vi "Settings.vi"(8 "error in":errorcluster, 10 "Main":T4={"Heat"={"KPтерм"=8.0, "TNтерм"=12.0, "KPниз"=4.0, "TNниз"=8.0, "COM ADC"="", "COM Termex"="", "KPдд"=4.0, "TNдд"=8.0, "Multiper"=1.0}, "Расчёты"={"Vm0"=8.0, "aa"=8.0, "bb"=8.0, "K0"=8.0, "A"=8.0, "B"=8.0}, "Видеосистема"=FALSE, "Anton Paar"={"IP adress"="192.168.0.110"}, "MIDA COM"="COM11"} caption="Настройки" {"Расчёты"."B" min=0.0 max=150.0 format="%.8f"; "Расчёты"."A" min=0.0 max=150.0 format="%.8f"; "Расчёты"."K0" min=0.0 max=150.0 format="%.2f"; "Расчёты"."bb" min=0.0 max=150.0 format="%.8f"; "Расчёты"."aa" min=0.0 max=150.0 format="%.8f"; "Расчёты"."Vm0" min=0.0 max=150.0 format="%.2f"; "Heat"."Multiper" min=0.0 max=150.0 format="%.2f"; "Heat"."TNдд" min=0.0 max=150.0 format="%.2f"; "Heat"."KPдд" min=0.0 max=150.0 format="%.2f"; "Heat"."TNниз" min=0.0 max=150.0 format="%.2f"; "Heat"."KPниз" min=0.0 max=150.0 format="%.2f"; "Heat"."TNтерм" min=0.0 max=150.0 format="%.2f"; "Heat"."KPтерм" min=0.0 max=150.0 format="%.2f"}) -> (0 "error out":errorcluster)   [LabVIEW 2023, in "Settings Master.lvlib"]
doc: "_____\nCreated using DQMH Event Scripter 6.1.0.128."
uses:
  Settings Master.lvlib
  Heat UI/Settings Type.ctl
  Drive/Calc_Type.ctl
  Menu/Setts.ctl
  Settings Argument--cluster.ctl
  Heat UI/Heat UI.lvlib
  Drive/Drive.lvlib
  Menu/Menu.lvlib
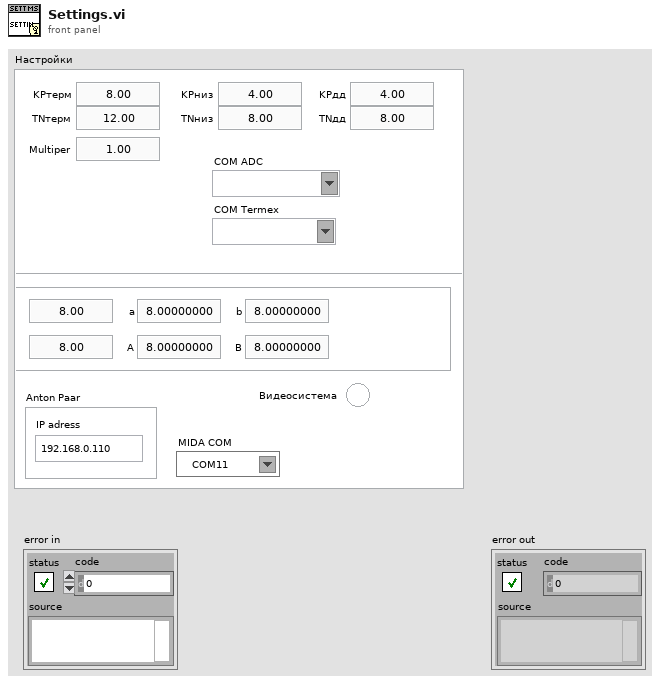
[diagram p1: front panel]
types:
  T1 = typedef "Heat UI.lvlib/Settings Type.ctl" = cluster{"KPтерм":dbl, "TNтерм":dbl, "KPниз":dbl, "TNниз":dbl, "COM ADC":refnum<visa-resource-name>, "COM Termex":refnum<visa-resource-name>, "KPдд":dbl, "TNдд":dbl, "Multiper":dbl}
  T2 = typedef "Drive.lvlib/Calc_Type.ctl" = cluster{"Vm0":dbl, "aa":dbl, "bb":dbl, "K0":dbl, "A":dbl, "B":dbl}
  T3 = typedef "Menu.lvlib/Setts.ctl" = cluster{"IP adress":string}
  T4 = cluster{"Heat":T1, "Расчёты":T2, "Видеосистема":bool, "Anton Paar":T3, "MIDA COM":refnum<visa-resource-name>}
  T5 = typedef "Settings Master.lvlib/Settings Argument--cluster.ctl" = cluster{"Main":cluster{"Heat":T1, "Расчёты":T2, "Видеосистема":bool, "Anton Paar":T3, "MIDA COM":refnum<visa-resource-name>}}
  T6 = typedef "Settings Master.lvlib/Broadcast Events--cluster.ctl" = cluster{"Module Did Init":refnum<user-event>, "Status Updated":refnum<user-event>, "Error Reported":refnum<user-event>, "Module Did Stop":refnum<user-event>, "Update Module Execution Status":refnum<user-event>, "Settings":refnum<user-event>}
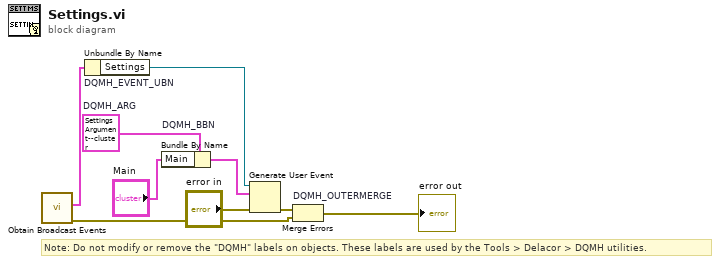
[diagram p0: block diagram]
diagram:
  w4 = T5 {"Main"={"Heat"={"KPтерм"=8.0, "TNтерм"=12.0, "KPниз"=4.0, "TNниз"=8.0, "COM ADC"="", "COM Termex"="", "KPдд"=4.0, "TNдд"=8.0, "Multiper"=1.0}, "Расчёты"={"Vm0"=8.0, "aa"=8.0, "bb"=8.0, "K0"=8.0, "A"=8.0, "B"=8.0}, "Видеосистема"=FALSE, "Anton Paar"={"IP adress"="192.168.0.110"}, "MIDA COM"="COM11"}}  # DQMH_ARG
  # "Note: Do not modify or remove the \"DQMH\" labels on objects. These labels are used by the Tools > Delacor > DQMH utilities."
  n1 = call "Obtain Broadcast Events.vi"() -> ("error out"=w2:errorcluster, "Settings Master Broadcast Events"=w1:T6)  [unwired: 10 in]
  n2 = Unbundle By Name "DQMH_EVENT_UBN"(w1) -> ("Settings"=w6:refnum<user-event>)
  n3 = Bundle By Name "DQMH_BBN"(cluster=w4, "Main"="Main") -> (w7:T5)
  n4 = Generate User Event(user event=w6, event data cluster=w7, error in="error in") -> (error out=w5:errorcluster)  [unwired: 1 in, 1 out]
  n5 = Merge Errors "DQMH_OUTERMERGE"(w5, w2) -> (→"error out":errorcluster)
